vi "DockMainPanel.vi"(8 "Error In":errorcluster, 11 "reference in":refnum<class "MasterGUI.lvclass">) -> (0 "Error Out":errorcluster, 3 "reference in":refnum<class "MasterGUI.lvclass">)   [LabVIEW 2021, in "MasterGUI.lvclass"]
uses:
  MasterGUI.lvclass
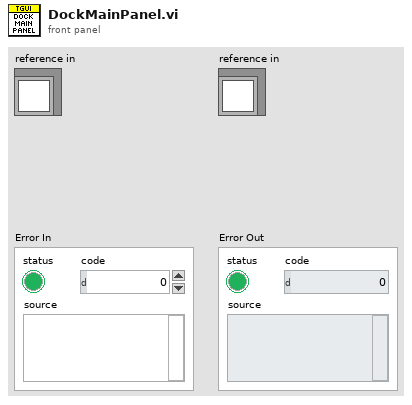
[diagram p1: front panel]
types:
  T1 = typedef "MasterGUI.lvclass/ObjectAttributes.ctl" = cluster{"Interfaces":cluster{"dummy":refnum<class>}, "Locals":cluster{"MainGUIActive":refnum<queue>, "MainPanel":refnum<vi>, "LayoutPanel":cluster{"PanelVIRef":refnum<vi>, "Labels":string[], "SubPanels":refnum<vi>[]}, "MenuTree":T2[], "Menu":refnum<k9>}, "Persistent":cluster{"StaticDocking":cluster{"ObjectLabel":string, "SubPanelLabel":string}[], "WindowsTitle":string, "AdditionalMenuItems":T2[], "TraceObjectName":string}}
  T2 = typedef "MasterGUI.lvclass/MenuItem.ctl" = cluster{"Parent":string, "Items":string[], "ShortCuts":cluster{"IncludeShiftKey":bool, "IncludeCtrlKey":bool, "ShortcutKey":string}[]}
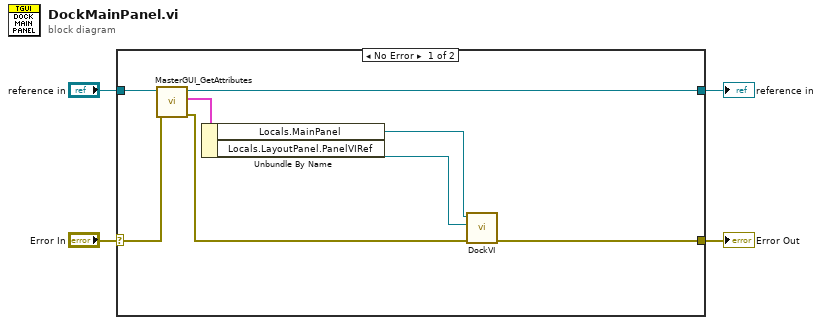
[diagram p0: block diagram]
diagram:
  n1 = case shown="No Error" "Error In" {
    selector: "Error In" -> [w12 w14]
    tunnel: [w8 w14] -> w3
    tunnel: [w9 w13] -> w1
    tunnel: "reference in" -> [w10 w13]
    frame No Error {
      n2 = call "MasterGUI_GetAttributes.vi"("error in (no error)"=w12, "reference in"=w10) -> ("error out"=w5:errorcluster, "Data"=w11:T1, "reference out"=w9:refnum<class "MasterGUI.lvclass">)  [unwired: 6 in, 1 out]
      n3 = Unbundle By Name(w11) -> ("Locals.MainPanel"=w7:refnum<vi>, "Locals.LayoutPanel.PanelVIRef"=w6:refnum<vi>)
      n4 = call "DockVI.vi"("error in (no error)"=w5, "PanelVIRef"=w6, "SubPanel in"=w7) -> ("error out"=w8:errorcluster)  [unwired: 8 in]
    }
    frame Error {
    }
  }
  "Error Out" <- w3
  "reference in" <- w1
